vi "Add Connection to State.vi"(8 "error in (no error)":errorcluster, 9 "Connection":T1, 10 "State":string, 11 "Channel Ref in":T2 format="%.0x") -> (0 "error out":errorcluster, 3 "Channel Ref out":T2=18446744073709551615 format="%.0x")   [LabVIEW 2017, in "Switch Scripting.lvlib"]
uses:
  Switch Scripting.lvlib
  <vilib>/NI Veristand/Custom Device API/Custom Device Item Ref.ctl
  Connection.ctl
  NationalInstruments.VeriStand.SystemDefinitionAPI
  Scripting Constants.vi
  <vilib>/NI VeriStand/Custom Device API/Custom Device API.lvlib
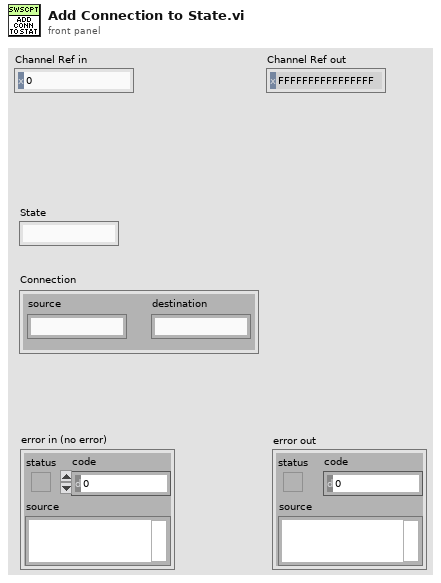
[diagram p1: front panel]
types:
  T1 = typedef "Switch Scripting.lvlib/Connection.ctl" = cluster{"source":string, "destination":string}
  T2 = typedef "Custom Device API.lvlib/Custom Device Item Ref.ctl" = u64
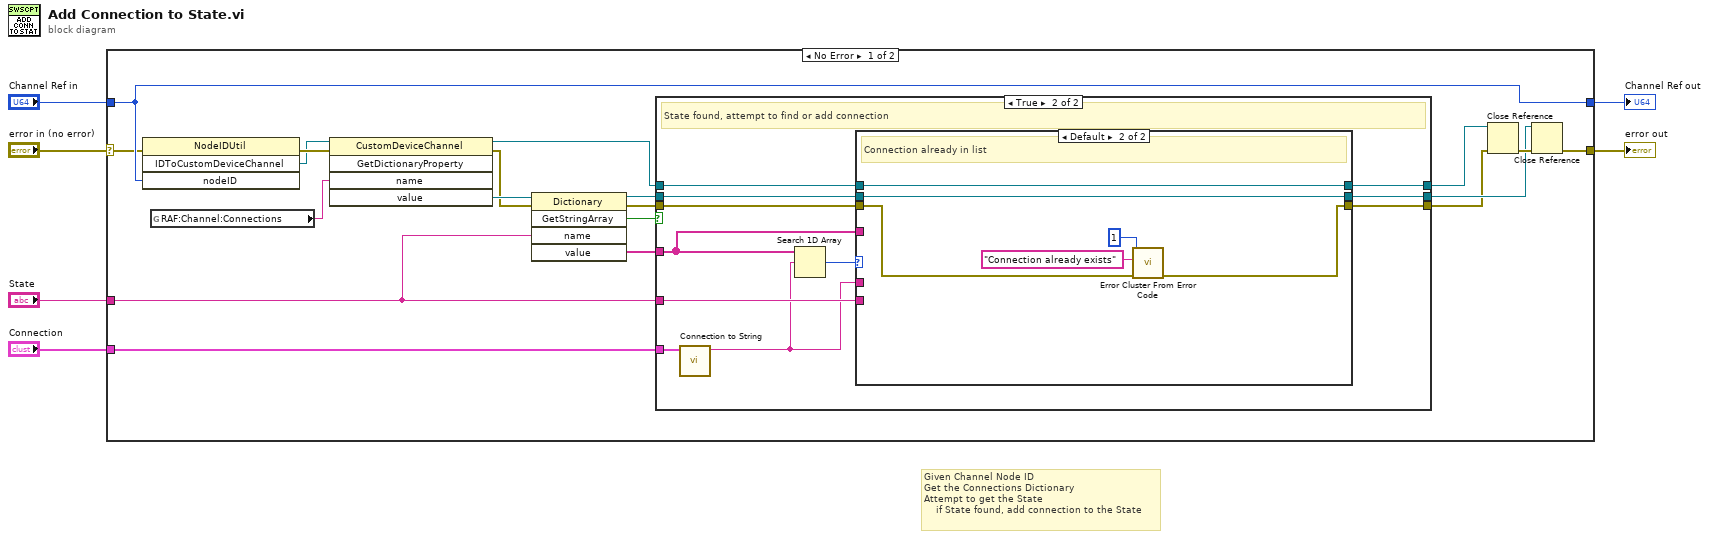
[diagram p0: block diagram]
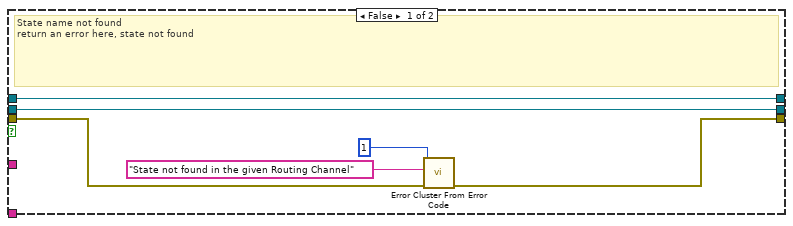
[diagram p2: hidden frame]
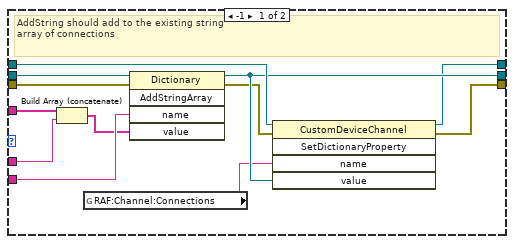
[diagram p3: hidden frame]
diagram:
  # "Given Channel Node ID\nGet the Connections Dictionary\nAttempt to get the State\n    if State found, add connection to the State"
  n1 = case shown="No Error" "error in (no error)" {
    selector: "error in (no error)" -> [w21 w62]
    tunnel: [w25 w62] -> w5
    tunnel: "Channel Ref in" -> [w22 w61]
    tunnel: [w22 w61] -> w3
    tunnel: "State" -> [w14 _]
    tunnel: "Connection" -> [w9 _]
    frame No Error {
      n2 = invoke class="NodeIDUtil" method="IDToCustomDeviceChannel"(error in=w21, "nodeID"=w22) -> (error out=w23:errorcluster, "IDToCustomDeviceChannel"=w11:refnum<k24>)  [unwired: 2 in, 2 out]
      n3 = global read "Scripting Constants.vi" "RAF:Channel:Connections"() -> (w8:string)
      n4 = invoke class="CustomDeviceChannel" method="GetDictionaryProperty"(reference=w11, error in=w23, "name"=w8) -> (reference out=w7:refnum<k24>, error out=w18:errorcluster, "value"=w19:refnum<k24>)  [unwired: 2 in, 2 out]
      n5 = invoke class="Dictionary" method="GetStringArray"(reference=w19, error in=w18, "name"=w14) -> (reference out=w15:refnum<k24>, error out=w16:errorcluster, "GetStringArray"=w17:bool, "value"=w20:string[])  [unwired: 2 in, 1 out]
      n6 = case shown="True" w17 {
        tunnel: w20 -> [_ w34]
        tunnel: w16 -> [w26 w41]
        tunnel: [w29 w40] -> w12
        tunnel: w14 -> [_ w39]
        tunnel: w15 -> [w28 w38]
        tunnel: [w28 w37] -> w13
        tunnel: w7 -> [w27 w36]
        tunnel: [w27 w35] -> w10
        tunnel: w9 -> [_ w33]
        frame False {
          # "State name not found\nreturn an error here, state not found"
          n7 = call <vilib>:"Error Cluster From Error Code.vi"("error in (no error)"=w26, "error message (\"\")"="State not found in the given Routing Channel" ("error message (\"\")"), "error code (0)"=1) -> ("error out"=w29:errorcluster)  [unwired: 6 in]
        }
        frame True {
          # "State found, attempt to find or add connection"
          n8 = call "Connection to String.vi"("Connection"=w33) -> ("String"=w32:string)  [unwired: 10 in]
          n9 = Search 1D Array(1D array=w34, element=w32) -> (index of element=w42:i32)  [unwired: 1 in]
          n10 = case shown="Default" w42 {
            tunnel: w41 -> [w52 w58]
            tunnel: [w48 w57] -> w40
            tunnel: w39 -> [w54 _]
            tunnel: w38 -> [w53 w56]
            tunnel: [w50 w56] -> w37
            tunnel: w36 -> [w51 w55]
            tunnel: [w47 w55] -> w35
            tunnel: w34 -> [w46 _]
            tunnel: w32 -> [w45 _]
            frame -1 {
              # "AddString should add to the existing string\narray of connections"
              n11 = Build Array (concatenate)(w46, w45) -> (w44:string[])
              n12 = global read "Scripting Constants.vi" "RAF:Channel:Connections"() -> (w43:string)
              n13 = invoke class="Dictionary" method="AddStringArray"(reference=w53, error in=w52, "name"=w54, "value"=w44) -> (reference out=w50:refnum<k24>, error out=w49:errorcluster)  [unwired: 1 in, 3 out]
              n14 = invoke class="CustomDeviceChannel" method="SetDictionaryProperty"(reference=w51, error in=w49, "name"=w43, "value"=w50) -> (reference out=w47:refnum<k24>, error out=w48:errorcluster)  [unwired: 1 in, 3 out]
            }
            frame Default {
              # "Connection already in list"
              n15 = call <vilib>:"Error Cluster From Error Code.vi"("error in (no error)"=w58, "error message (\"\")"="Connection already exists" ("error message (\"\")"), "error code (0)"=1) -> ("error out"=w57:errorcluster)  [unwired: 6 in]
            }
          }
        }
      }
      n16 = Close Reference(reference=w10, error in (no error)=w12) -> (error out=w24:errorcluster)
      n17 = Close Reference(reference=w13, error in (no error)=w24) -> (error out=w25:errorcluster)
    }
    frame Error {
    }
  }
  "Channel Ref out" <- w3
  "error out" <- w5
